vi "array n 2 to 1.vi"(11 "2N array":dbl[][](array[numeric])) -> (3 "1N array":dbl[](array[numeric]))   [LabVIEW 2018]
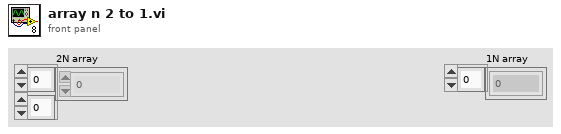
[diagram p1: front panel]
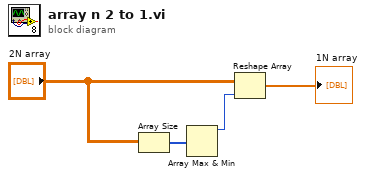
[diagram p0: block diagram]
diagram:
  n1 = Array Size(array="2N array") -> (size(s)=w3:i32[])
  n2 = Array Max & Min(array=w3) -> (max value=w2:i32)  [unwired: 3 out]
  n3 = Reshape Array("2N array", w2) -> (→"1N array":dbl[])
